vi "GT_GetCaptureStatus.vi"(9 "count":i16, 10 "encode":i16, 11 "rtn_In":cluster{"rtn":i16, "Func":string}) -> (0 "Status":bool, 1 "pStatus":i16, 2 "encode out":i16, 3 "rtn_Out":cluster{"rtn":i16, "Func":string}, 5 "pValue":i32)   [LabVIEW 2014]
uses:
  VC6/gts.dll
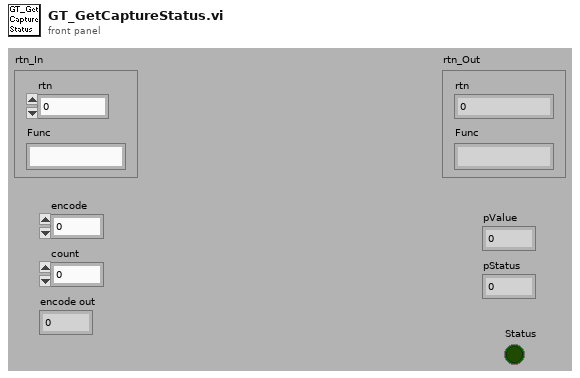
[diagram p1: front panel]
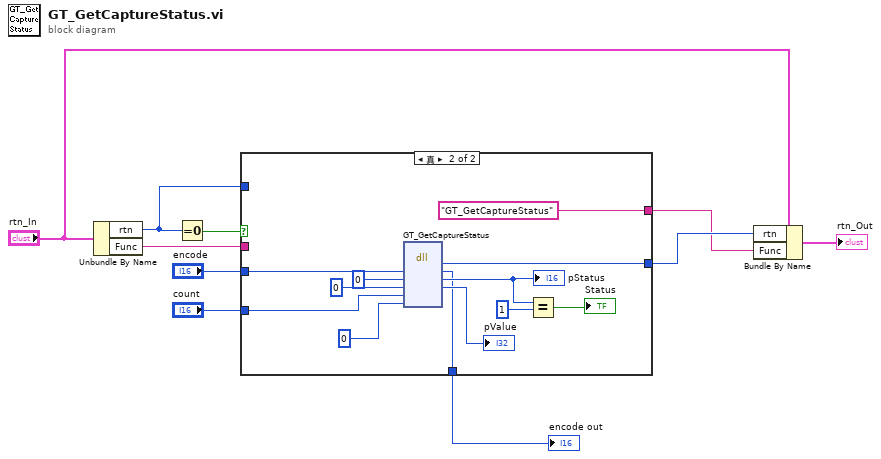
[diagram p0: block diagram]
diagram:
  n1 = Unbundle By Name("rtn_In") -> ("rtn"=w3:i16, "Func"=w2:string)
  n2 = Equal To 0?(x=w3) -> (x = 0?=w10:bool)
  n3 = case shown="真" w10 {
    tunnel: [w13 w25] -> w7
    tunnel: [w12 "GT_GetCaptureStatus" ("Func")] -> w6
    tunnel: "encode" -> [w11 w23]
    tunnel: "count" -> [_ w22]
    tunnel: w3 -> [w13 _]
    tunnel: w2 -> [w12 _]
    tunnel: [w11 w15] -> w1
    frame False {
    }
    frame True {
      n4 = dll-call lib="PTH2Fabs DNewGTS AC-800LWin7版源程序-20170926gts85VC6gts.dll" fn="GT_GetCaptureStatus"("encode"=w23, "pStatus"=i16 0, "pValue"=0, "count"=w22, "pClock"=u32 0) -> ("rtn"=w25:i16, "encode"=w15:i16, "pStatus"=w18:i16, "pValue"=→"pValue":i32)  [unwired: 5 in, 2 out]
      "pStatus" <- w18
      n5 = Equal?(x=w18, y=i16 1) -> (x = y?=→"Status":bool)
    }
  }
  "encode out" <- w1
  n6 = Bundle By Name(cluster="rtn_In", "rtn"=w7, "Func"=w6) -> (→"rtn_Out":cluster{"rtn":i16, "Func":string})
